vi "Data_MultiDisplayMode.vi"(0 "taskHandle":variant, 1 "wfm info":T1, 2 "wfm info 2":T1, 3 "显示方式":u16(ring) items=["原始显示", "拆分显示"], 5 "taskHandle 2":variant, 7 "1D data":dbl[](array[numeric]), 9 "1D data 2":dbl[](array[numeric]), 11 "error in":errorcluster, 12 "displayLength":u32) -> (8 "2D data":dbl[][](array[numeric]), 15 "error out":errorcluster)   [LabVIEW 2013]
uses:
  <userlib>/ArtScope/_SubVI/ArtScope_ArrayByChannel_DBL.vi
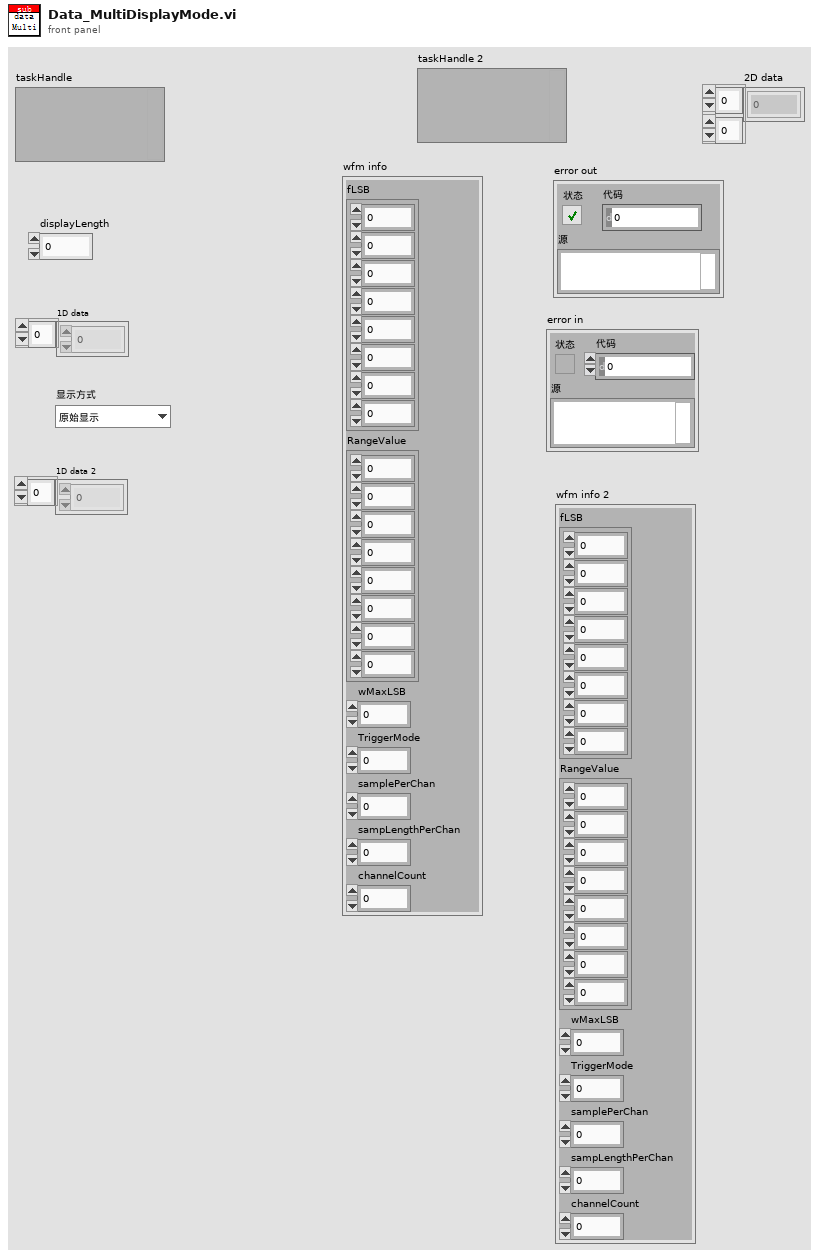
[diagram p1: front panel]
types:
  T1 = cluster{"fLSB":cluster{dbl, dbl, dbl, dbl, dbl, dbl, dbl, dbl}, "RangeValue":cluster{dbl, dbl, dbl, dbl, dbl, dbl, dbl, dbl}, "wMaxLSB":u32, "TriggerMode":i32, "samplePerChan":u32, "sampLengthPerChan":u32, "channelCount":i32}
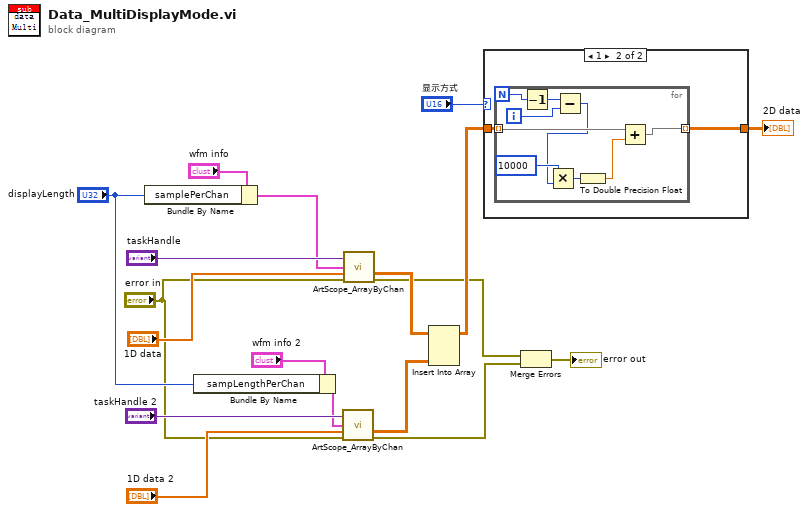
[diagram p0: block diagram]
diagram:
  n1 = Bundle By Name(cluster="wfm info", "samplePerChan"="displayLength") -> (w16:T1)
  n2 = Bundle By Name(cluster="wfm info 2", "sampLengthPerChan"="displayLength") -> (w9:T1)
  n3 = call-poly <userlib>:"ArtScope_ArrayByChan.vi"("task handle"="taskHandle 2", "wfm info"=w9, "1D data"="1D data 2", "error in (no error)"="error in") -> ("2D data"=w7:dbl[][], "error out"=w4:errorcluster)  [unwired: 9 in, 1 out]
  n4 = call-poly <userlib>:"ArtScope_ArrayByChan.vi"("task handle"="taskHandle", "wfm info"=w16, "1D data"="1D data", "error in (no error)"="error in") -> ("2D data"=w8:dbl[][], "error out"=w5:errorcluster)  [unwired: 9 in, 1 out]
  n5 = Insert Into Array(array=w8, new element=w7) -> (w6:dbl[][])  [unwired: 2 in]
  n6 = case shown="1" "显示方式" {
    tunnel: w6 -> [w19 w21]
    tunnel: [w19 w20] -> w13
    frame 0, Default {
    }
    frame 1 {
      n7 = for {
        N -> [w25]
        tunnel: w21 -> [w30] mode=indexing
        tunnel: [w26] -> w20 mode=indexing
        i -> [w23]
        n8 = Decrement(x=w25) -> (x-1=w24:i32)
        n9 = Subtract(x=w24, y=w23) -> (x-y=w22:i32)
        n10 = Multiply(x=10000, y=w22) -> (x*y=w28:i32)
        n11 = To Double Precision Float(number=w28) -> (double precision float=w27:dbl)
        n12 = Add(x=w30, y=w27) -> (x+y=w26:dbl[])
      }
    }
  }
  "2D data" <- w13
  n13 = Merge Errors(w5, w4) -> (→"error out":errorcluster)
